vi "Define_dR_Area_for_Problem_Point-3.vi"(4 "[IN] Areas particles\nPrimary Detected":dbl[][](array[numeric]), 6 "[IN] Primary \n(X,Y) Detected":dbl[][](array[numeric]), 8 "error IN":errorcluster, 9 "[IN] Subtrack":T1) -> (0 "error OUT":errorcluster, 2 "[OUT] Area Problem Point\n101 - Starting Point\n11 - Ending Point":dbl, 3 "[OUT] dR for Problem Point":dbl)   [LabVIEW 2013]
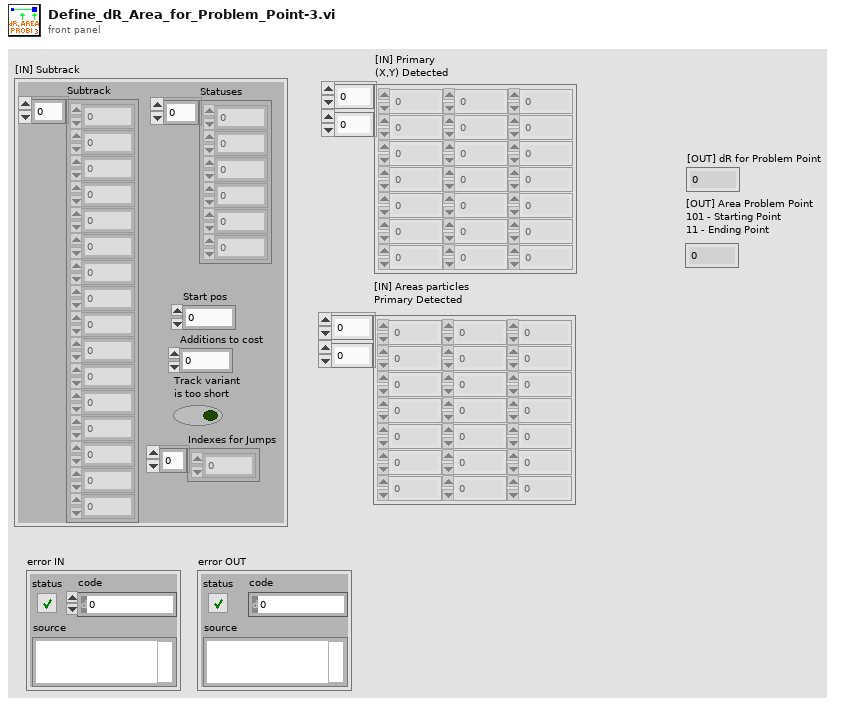
[diagram p1: front panel]
types:
  T1 = cluster{"Subtrack":dbl[], "Statuses":i16[], "Start pos":i32, "Additions to cost":i8, "Track variant \nis too short":bool, "Indexes for Jumps":i32[]}
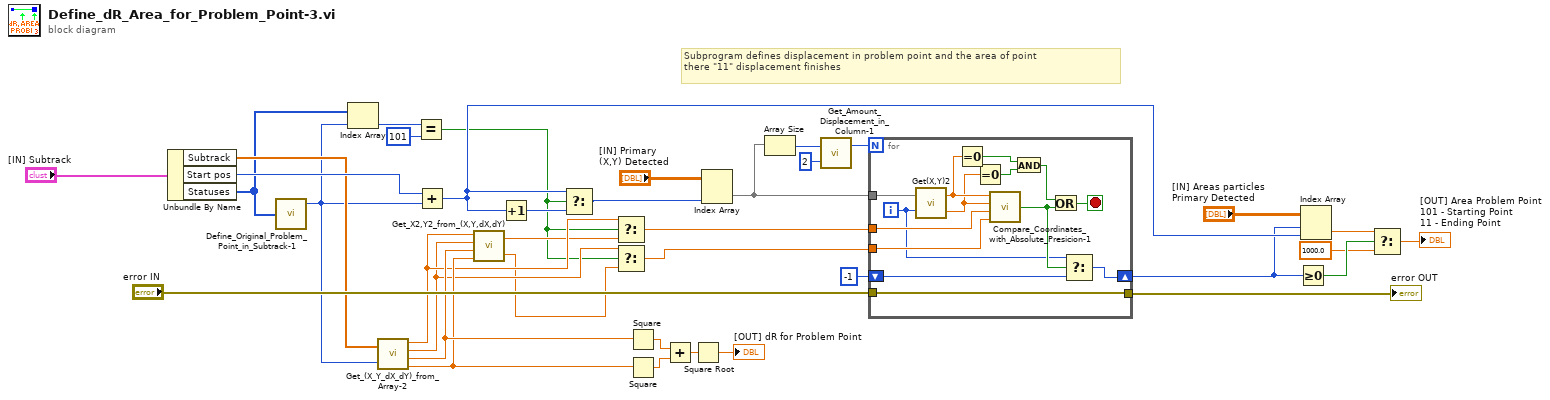
[diagram p0: block diagram]
diagram:
  # "Subprogram defines displacement in problem point and the area of point \nthere \"11\" displacement finishes"
  n1 = Unbundle By Name("[IN] Subtrack") -> ("Subtrack"=w20:dbl[], "Start pos"=w27:i32, "Statuses"=w19:i16[])
  n2 = call "Define_Original_Problem_Point_in_Subtrack-1.vi"("[IN] Statuses"=w19) -> ("[OUT] Index of Problem Point\nin Subtrack (Original)"=w18:i32)  [unwired: 3 in, 1 out]
  n3 = Index Array(array=w19, index=w18) -> (element=w17:i16)
  n4 = call "Get_(X_Y_dX_dY)_from_Array-2.vi"("(X,Y,dX,dY)"=w20, "Index of Displacement"=w18) -> ("X"=w12:dbl, "Y"=w9:dbl, "dX"=w22:dbl, "dY"=w21:dbl)
  n5 = Equal?(x=w17, y=i16 101) -> (x = y?=w8:bool)
  n6 = Add(x=w27, y=w18) -> (x+y=w15:i32)
  n7 = call "Get_X2,Y2_from_(X,Y,dX,dY).vi"("dY"=w21, "dX"=w22, "Y1"=w9, "X1"=w12) -> ("Y2 = (Y1+dY)"=w7:dbl, "X2 = (X1+dX)"=w11:dbl)
  n8 = Increment(x=w15) -> (x+1=w14:i32)
  n9 = Select(t=w15, s=w8, f=w14) -> (s? t:f=w13:i32)
  n10 = Select(t=w12, s=w8, f=w11) -> (s? t:f=w10:dbl)
  n11 = Select(t=w9, s=w8, f=w7) -> (s? t:f=w6:dbl)
  n12 = Square(x=w22) -> (x^2=w36:dbl)
  n13 = Square(x=w21) -> (x^2=w35:dbl)
  n14 = Add(x=w36, y=w35) -> (x+y=w34:dbl)
  n15 = Square Root(x=w34) -> (sqrt(x)=→"[OUT] dR for Problem Point":dbl)
  n16 = Index Array(array="[IN] Primary \n(X,Y) Detected", index (col)=w13) -> (element=w28:dbl[])  [unwired: 1 in]
  n17 = Array Size(array=w28) -> (size(s)=w32:i32)
  n18 = call "Get_Amount_Displacement_in_Column-1.vi"("multiplier"=2, "# Rows"=w32) -> ("Displ amount"=w30:i32)  [unwired: 1 out]
  n19 = for {
    N: w30 -> [_]
    tunnel: w28 -> [w50]
    tunnel: w10 -> [w49]
    tunnel: w6 -> [w48]
    shift-right: [w39] -> w5
    shift-left: -1 -> [w40]
    tunnel: "error IN" -> [w38]
    tunnel: [w38] -> w24
    i -> [w41]
    stop <- w51 stop-if-true
    n20 = call "Get(X,Y)2.vi"("[IN] index of (X,Y)"=w41, "[IN] Array coordi\nnates (X,Y) in Frame"=w50) -> ("[OUT] Y"=w44:dbl, "[OUT] X"=w45:dbl)
    n21 = Equal To 0?(x=w45) -> (x = 0?=w47:bool)
    n22 = Equal To 0?(x=w44) -> (x = 0?=w46:bool)
    n23 = call "Compare_Coordinates_with_Absolute_Presicion-1.vi"("X 1"=w45, "Y 1"=w44, "X 2"=w49, "Y 2"=w48) -> ("[OUT] Same coordinates?"=w42:bool)  [unwired: 1 in]
    n24 = And(x=w47, y=w46) -> (x .and. y?=w43:bool)
    n25 = Or(x=w43, y=w42) -> (x .or. y?=w51:bool)
    n26 = Select(t=w41, s=w42, f=w40) -> (s? t:f=w39:i32)
  }
  "error OUT" <- w24
  n27 = Greater Or Equal To 0?(x=w5) -> (x >= 0?=w4:bool)
  n28 = Index Array(array="[IN] Areas particles\nPrimary Detected", index (row)=w5, index (col)=w15) -> (element=w3:dbl)
  n29 = Select(t=w3, s=w4, f=1000.0) -> (s? t:f=→"[OUT] Area Problem Point\n101 - Starting Point\n11 - Ending Point":dbl)
